vi "Generate.vi"(8 "error in (no error)":errorcluster, 11 "Sine in":refnum<class "Sine.lvclass">) -> (0 "error out":errorcluster, 3 "Sine out":refnum<class "Sine.lvclass">)   [LabVIEW 2020, in "Sine.lvclass"]
uses:
  Sine.lvclass
  C:/Users/fflores/Documents/GitHub Projects/OOP-Concepts-in-LabVIEW/Design Patterns/Composite Pattern/Analog Waveform/Analog Waveform.lvclass
  <vilib>/measure/NI_MABase.lvlib
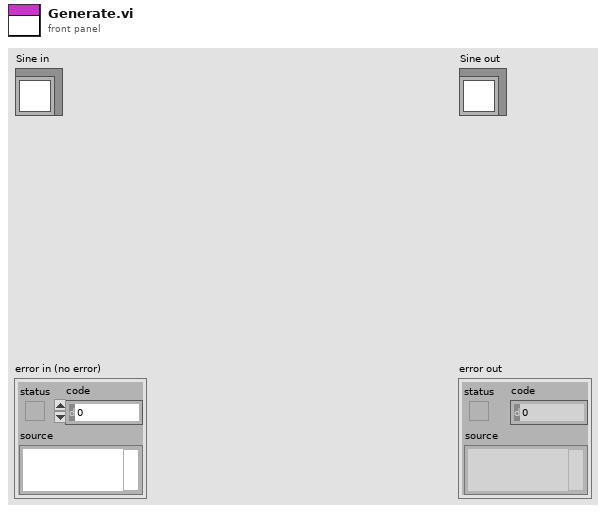
[diagram p1: front panel]
types:
  T1 = enum16{"Sine Wave", "Triangle Wave", "Square Wave", "Sawtooth Wave"}
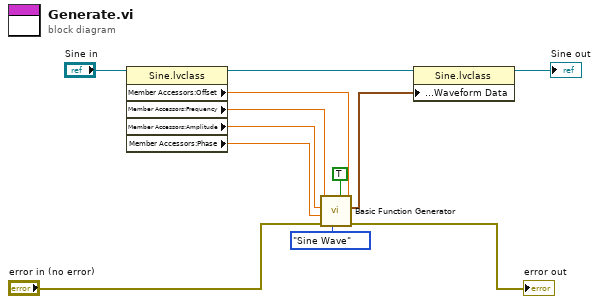
[diagram p0: block diagram]
diagram:
  n1 = property class="Sine.lvclass"(reference="Sine in") -> (reference out=w11:refnum<class "Sine.lvclass">, "Member Accessors:Offset"=w10:dbl, "Member Accessors:Frequency"=w9:dbl, "Member Accessors:Amplitude"=w8:dbl, "Member Accessors:Phase"=w7:dbl)  [unwired: 1 in, 1 out]
  n2 = call <vilib>:"Basic Function Generator.vi"("offset"=w10, "reset signal"=TRUE, "signal type"=T1."Sine Wave", "error in (no error)"="error in (no error)", "phase"=w7, "amplitude"=w8, "frequency"=w9) -> ("error out"=→"error out":errorcluster, "signal out"=w2:waveform(dbl))  [unwired: 2 in, 1 out]
  n3 = property class="Sine.lvclass"(reference=w11, "Member Accessors:Waveform Data"=w2) -> (reference out=→"Sine out":refnum<class "Sine.lvclass">)  [unwired: 1 in, 1 out]
